vi "Inset To Table.vi"(8 "Column Size":i32=-1, 9 "Paste Value":string[](array[string]), 10 "Selection Start":T1, 11 "Table Value":string[][](array[string])) -> (3 "1D String Out":string[](array[string]))   [LabVIEW 2024]
uses:
  <vilib>/Utility/miscctls.llb/LVRowAndColumnTypeDef.ctl
  Converter/String Trimming 2D to 1D.vi
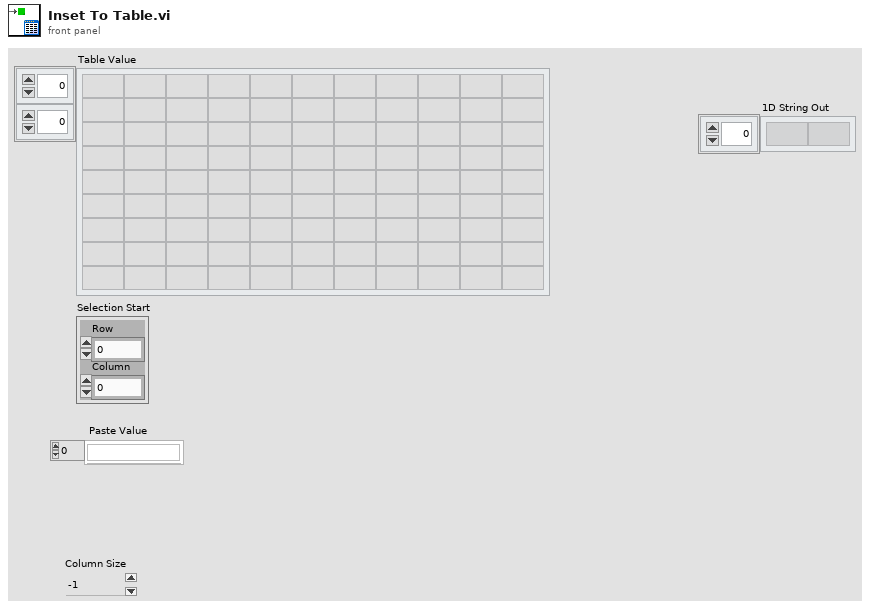
[diagram p1: front panel]
types:
  T1 = typedef "LVRowAndColumnTypeDef.ctl" = cluster{"Row":i32, "Column":i32}
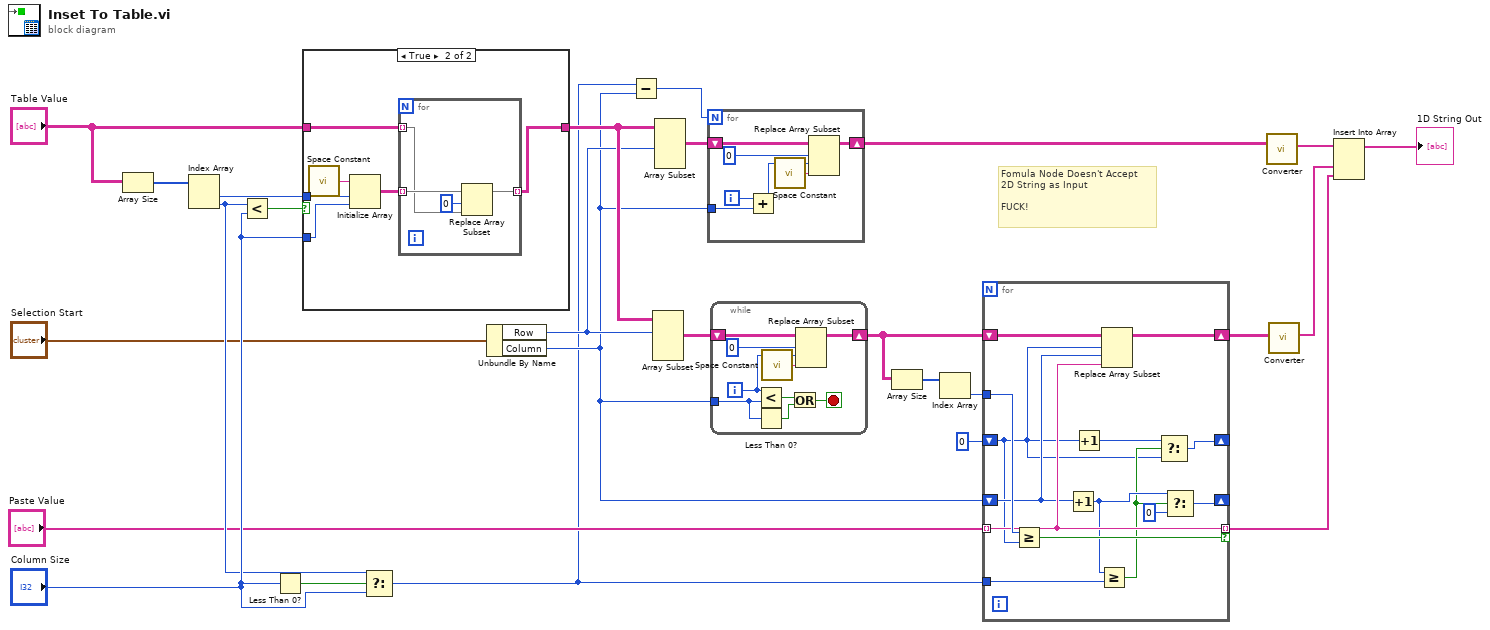
[diagram p0: block diagram]
diagram:
  # "Fomula Node Doesn't Accept \n2D String as Input\n\nFUCK!"
  n1 = Array Size(array="Table Value") -> (size(s)=w26:i32[])
  n2 = Index Array(array=w26) -> (element #1=w23:i32, element #2=w20:i32)  [unwired: 2 in]
  n3 = Less?(x=w20, y="Column Size") -> (x < y?=w25:bool)
  n4 = Less Than 0?(x="Column Size") -> (x < 0?=w22:bool)
  n5 = case shown="True" w25 {
    tunnel: "Table Value" -> [w27 w29]
    tunnel: w23 -> [_ w33]
    tunnel: "Column Size" -> [_ w31]
    tunnel: [w27 w28] -> w18
    frame False {
    }
    frame True {
      n6 = call <vilib>:"Space Constant.vi"() -> ("String"=w32:string)
      n7 = Initialize Array(w32, w33, w31) -> (w30:string[][])
      n8 = for {
        tunnel: w30 -> [w37] mode=indexing
        tunnel: w29 -> [w36] mode=indexing
        tunnel: [w34] -> w28 mode=indexing
        n9 = Replace Array Subset(array=w37, new element=w36, index=0) -> (w34:string[])
      }
    }
  }
  n10 = Select(t=w20, s=w22, f="Column Size") -> (s? t:f=w5:i32)
  n11 = Unbundle By Name("Selection Start") -> ("Row"=w17:i32, "Column"=w7:i32)
  n12 = Subtract(x=w5, y=w7) -> (x-y=w11:i32)
  n13 = Array Subset(array=w18, index (row)=w17) -> (w14:string[][])  [unwired: 3 in]
  n14 = Array Subset(array=w18, length (row)=w17) -> (w13:string[][])  [unwired: 3 in]
  n15 = for {
    N: w11 -> [_]
    shift-right: [w43] -> w12
    shift-left: w13 -> [w44]
    tunnel: w7 -> [w39]
    i -> [w40]
    n16 = Add(x=w40, y=w39) -> (x+y=w38:i32)
    n17 = call <vilib>:"Space Constant.vi"() -> ("String"=w42:string)
    n18 = Replace Array Subset(array=w44, new element=w42, index (row)=0, index (col)=w38) -> (w43:string[][])
  }
  n19 = while {
    tunnel: w7 -> [w48]
    shift-right: [w52] -> w4
    shift-left: w14 -> [w53]
    i -> [w49]
    stop <- w47 stop-if-true
    n20 = Less?(x=w49, y=w48) -> (x < y?=w46:bool)
    n21 = Less Than 0?(x=w48) -> (x < 0?=w45:bool)
    n22 = call <vilib>:"Space Constant.vi"() -> ("String"=w51:string)
    n23 = Or(x=w46, y=w45) -> (x .or. y?=w47:bool)
    n24 = Replace Array Subset(array=w53, new element=w51, index (row)=0, index (col)=w49) -> (w52:string[][])
  }
  n25 = Array Size(array=w4) -> (size(s)=w3:i32[])
  n26 = Index Array(array=w3) -> (element=w2:i32)  [unwired: 1 in]
  n27 = for {
    shift-right: [w64] -> w10
    shift-left: w4 -> [w65]
    tunnel: "Paste Value" -> [w63] mode=indexing
    shift-right: [w57] -> _
    shift-left: 0 ("Column") -> [w55]
    shift-right: [w59] -> _
    shift-left: w7 -> [w62]
    tunnel: w5 -> [w61]
    tunnel: w2 -> [w67]
    tunnel: [w63] -> w1 mode=indexing if=w66
    n28 = Greater Or Equal?(x=w67, y=w55) -> (x >= y?=w66:bool)
    n29 = Increment(x=w62) -> (x+1=w60:i32)
    n30 = Increment(x=w55) -> (x+1=w54:i32)
    n31 = Greater Or Equal?(x=w60, y=w61) -> (x >= y?=w56:bool)
    n32 = Replace Array Subset(array=w65, new element=w63, index (row)=w55, index (col)=w62) -> (w64:string[][])
    n33 = Select(t=w54, s=w56, f=w55) -> (s? t:f=w57:i32)
    n34 = Select(t=w60, s=w56, f=0) -> (s? t:f=w59:i32)
  }
  n35 = call-poly "Converter.vi"("1D String In"=w12) -> ("1D String Out"=w16:string[])  [unwired: 10 in]
  n36 = call-poly "Converter.vi"("1D String In"=w10) -> ("1D String Out"=w9:string[])  [unwired: 10 in]
  n37 = Insert Into Array(array=w16, new element #1=w9, new element #2=w1) -> (→"1D String Out":string[])  [unwired: 1 in]
